vi "from_guid.vi"(8 "error in (no error)":errorcluster, 10 "guid (\"\": generate new)":string, 11 "Node in":refnum<class "Node.lvclass">) -> (0 "error out":errorcluster, 3 "Node out":refnum<class "Node.lvclass">)   [LabVIEW 2020, in "graph.lvlib" / "Node.lvclass"]
uses:
  Node.lvclass
  Node.lvclass/Node.ctl
  ID/ID.lvclass
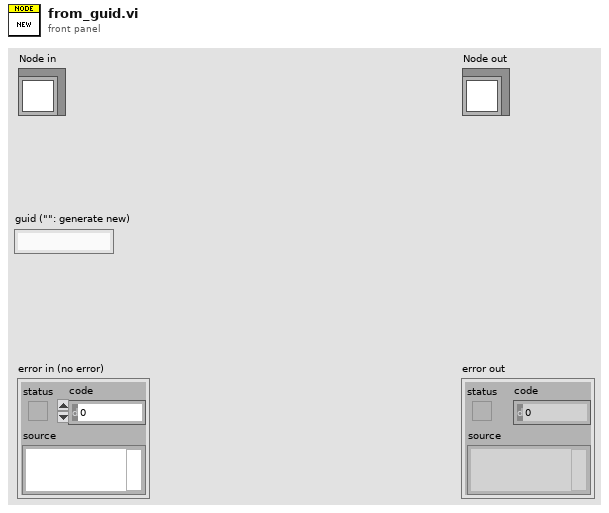
[diagram p1: front panel]
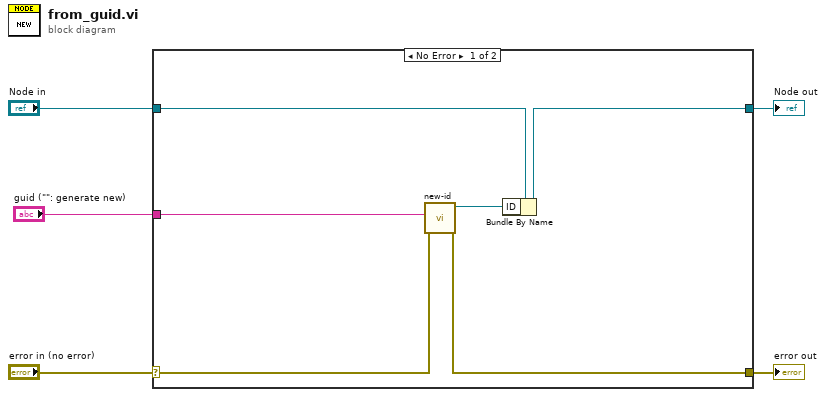
[diagram p0: block diagram]
diagram:
  n1 = case shown="No Error" "error in (no error)" {
    selector: "error in (no error)" -> [w8 w13]
    tunnel: [w7 w13] -> w4
    tunnel: [w10 w12] -> w2
    tunnel: "Node in" -> [w11 w12]
    tunnel: "guid (\"\": generate new)" -> [w6 _]
    frame No Error {
      n2 = call "new-id.vi"("error in (no error)"=w8, "id-string (\"\": generate new id)"=w6) -> ("error out"=w7:errorcluster, "ID out"=w9:refnum<class "ID.lvclass">)  [unwired: 8 in]
      n3 = Bundle By Name(cluster=w11, "ID"=w9) -> (w10:refnum<class "Node.lvclass">)
    }
    frame Error {
    }
  }
  "error out" <- w4
  "Node out" <- w2
